vi "TELEOP BUTTONS.vi"(10 "Joystick values":T1(array[cluster])) -> ()   [LabVIEW 2020]
uses:
  <vilib>/Rock Robotics/Network Tables/NT Read Boolean.vi
  <vilib>/Rock Robotics/Network Tables/NT Write Boolean.vi
  <vilib>/Rock Robotics/Network Tables/NT Read Number.vi
  <vilib>/Rock Robotics/Network Tables/NT Read Numeric Array.vi
  <vilib>/Rock Robotics/Network Tables/NT Write Number.vi
panel:
  in  "INTAKE ARM DOWN":cluster{"Joystick":u16, "BUTTON":i32}={"Joystick"=2, "BUTTON"=9} {"Joystick" items=["RIGHT TANK (default)", "LEFT ARM", "RIGHT ARM", "LEFT TANK DRIVE"]}
  in  "FIRE CARGO":cluster{"Joystick":u16, "BUTTON":i32} {"Joystick" items=["RIGHT TANK (default)", "LEFT ARM", "RIGHT ARM", "LEFT TANK DRIVE"]}
  in  "SHOOTER SPEEDS":u16(ring) items=["HI", "LO", "PUKE"]
  in  "SHOOTER off":cluster{"Joystick":u16, "BUTTON":i32}={"Joystick"=2, "BUTTON"=11} {"Joystick" items=["RIGHT TANK (default)", "LEFT ARM", "RIGHT ARM", "LEFT TANK DRIVE"]}
  in  "SHOOTER puke":cluster{"Joystick":u16, "BUTTON":i32}={"Joystick"=2, "BUTTON"=10} {"Joystick" items=["RIGHT TANK (default)", "LEFT ARM", "RIGHT ARM", "LEFT TANK DRIVE"]}
  in  "CLIMBER TURBO":cluster{"Joystick":u16, "BUTTON":i32}={"Joystick"=2, "BUTTON"=9} {"Joystick" items=["RIGHT TANK (default)", "LEFT ARM", "RIGHT ARM", "LEFT TANK DRIVE"]}
  in  "SHOOTER LO":cluster{"Joystick":u16, "BUTTON":i32}={"Joystick"=2, "BUTTON"=8} {"Joystick" items=["RIGHT TANK (default)", "LEFT ARM", "RIGHT ARM", "LEFT TANK DRIVE"]}
  in  "SHOOTER HI":cluster{"Joystick":u16, "BUTTON":i32}={"Joystick"=2, "BUTTON"=7} {"Joystick" items=["RIGHT TANK (default)", "LEFT ARM", "RIGHT ARM", "LEFT TANK DRIVE"]}
  in  "TOGGLE PAWL LOCKS":cluster{"Joystick":u16, "BUTTON":i32}={"Joystick"=2, "BUTTON"=6} {"Joystick" items=["RIGHT TANK (default)", "LEFT ARM", "RIGHT ARM", "LEFT TANK DRIVE"]}
  in  "MACRO LOW BAR CLIMB":cluster{"Joystick":u16, "BUTTON":i32}={"Joystick"=1, "BUTTON"=11} {"Joystick" items=["RIGHT TANK (default)", "LEFT ARM", "RIGHT ARM", "LEFT TANK DRIVE"]}
  in  "INTAKE rollers toggle ON/OFF":cluster{"Joystick":u16, "BUTTON":i32}={"Joystick"=1, "BUTTON"=10} {"Joystick" items=["RIGHT TANK (default)", "LEFT ARM", "RIGHT ARM", "LEFT TANK DRIVE"]}
  in  "INTAKE raise/lower":cluster{"Joystick":u16, "BUTTON":i32}={"Joystick"=1, "BUTTON"=9} {"Joystick" items=["RIGHT TANK (default)", "LEFT ARM", "RIGHT ARM", "LEFT TANK DRIVE"]}
  in  "MACRO overide":cluster{"Joystick":u16, "BUTTON":i32}={"Joystick"=1, "BUTTON"=6} {"Joystick" items=["RIGHT TANK (default)", "LEFT ARM", "RIGHT ARM", "LEFT TANK DRIVE"]}
  in  "MACRO step forward":cluster{"Joystick":u16, "BUTTON":i32}={"Joystick"=1, "BUTTON"=7} {"Joystick" items=["RIGHT TANK (default)", "LEFT ARM", "RIGHT ARM", "LEFT TANK DRIVE"]}
  in  "MACRO step back":cluster{"Joystick":u16, "BUTTON":i32}={"Joystick"=1, "BUTTON"=8} {"Joystick" items=["RIGHT TANK (default)", "LEFT ARM", "RIGHT ARM", "LEFT TANK DRIVE"]}
  in  "AXIS VALUES in":u16(ring) items=["X axis", "Y axis", "Z axis"]
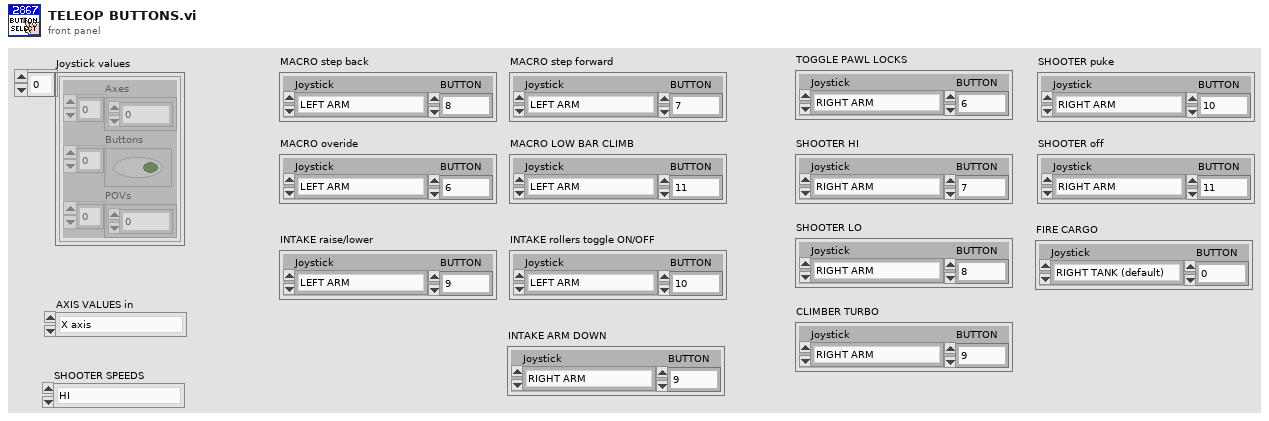
[diagram p1: front panel]
types:
  T1 = cluster{"Axes":dbl[], "Buttons":bool[], "POVs":i16[]}[]
  T2 = cluster{"SHOOTER HI":cluster{"Joystick":u16, "BUTTON":i32}, "SHOOTER puke":cluster{"Joystick":u16, "BUTTON":i32}, "CLIMBER TURBO":cluster{"Joystick":u16, "BUTTON":i32}, "MACRO overide":cluster{"Joystick":u16, "BUTTON":i32}, "TOGGLE PAWL LOCKS":cluster{"Joystick":u16, "BUTTON":i32}, "SHOOTER LO":cluster{"Joystick":u16, "BUTTON":i32}, "MACRO LOW BAR CLIMB":cluster{"Joystick":u16, "BUTTON":i32}, "MACRO step forward":cluster{"Joystick":u16, "BUTTON":i32}, "INTAKE rollers toggle ON/OFF":cluster{"Joystick":u16, "BUTTON":i32}, "MACRO step back":cluster{"Joystick":u16, "BUTTON":i32}, "INTAKE raise/lower":cluster{"Joystick":u16, "BUTTON":i32}, "SHOOTER off":cluster{"Joystick":u16, "BUTTON":i32}, "FIRE CARGO":cluster{"Joystick":u16, "BUTTON":i32}, "INTAKE ARM DOWN":cluster{"Joystick":u16, "BUTTON":i32}}
  T3 = cluster{"Axes":dbl[], "Buttons":bool[], "POVs":i16[]}
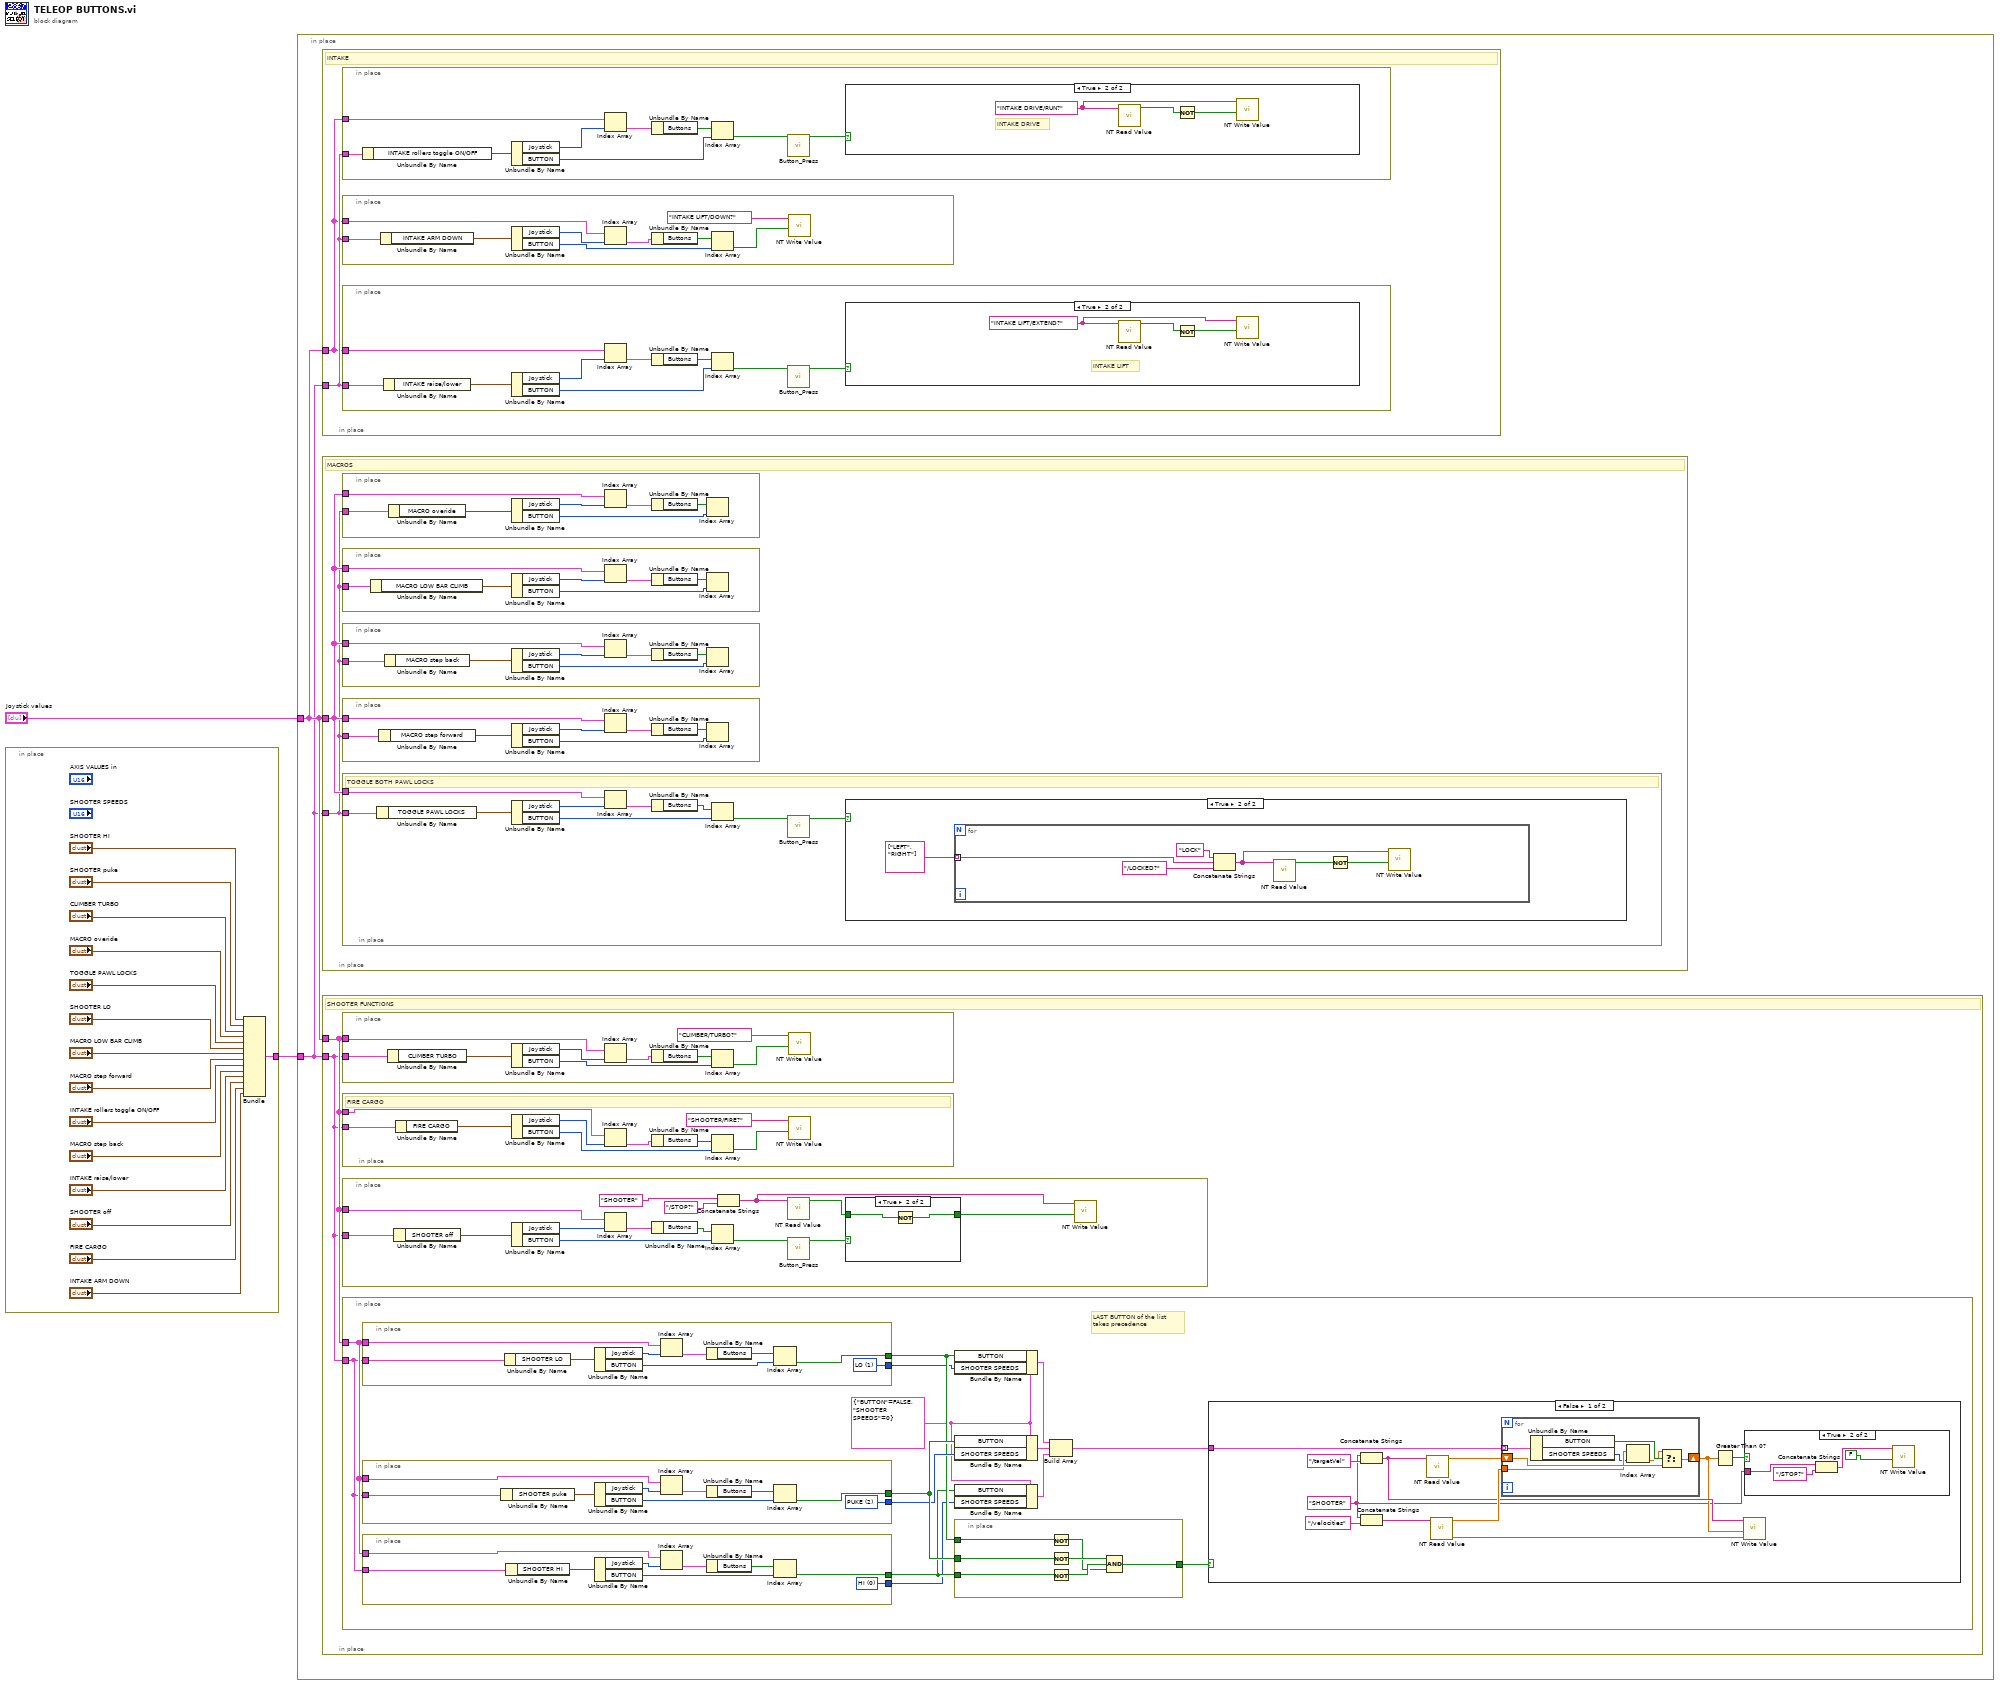
[diagram p0: block diagram]
diagram:
  n1 = in-place {
    in-place-border: [w6] -> w1
    n2 = Bundle("SHOOTER HI"="SHOOTER HI", "SHOOTER puke"="SHOOTER puke", "CLIMBER TURBO"="CLIMBER TURBO", "MACRO overide"="MACRO overide", "TOGGLE PAWL LOCKS"="TOGGLE PAWL LOCKS", "SHOOTER LO"="SHOOTER LO", "MACRO LOW BAR CLIMB"="MACRO LOW BAR CLIMB", "MACRO step forward"="MACRO step forward", "INTAKE rollers toggle ON/OFF"="INTAKE rollers toggle ON/OFF", "MACRO step back"="MACRO step back", "INTAKE raise/lower"="INTAKE raise/lower", "SHOOTER off"="SHOOTER off", "FIRE CARGO"="FIRE CARGO", "INTAKE ARM DOWN"="INTAKE ARM DOWN") -> (w6:T2)  [unwired: 1 in]
  }
  n3 = in-place {
    in-place-border: "Joystick values" -> [w19]
    in-place-border: w1 -> [w18]
    n4 = in-place {
      in-place-border: w19 -> [w173]
      in-place-border: w18 -> [w174]
      # "INTAKE"
      n5 = in-place {
        in-place-border: w173 -> [w192]
        in-place-border: w174 -> [w189]
        n6 = Unbundle By Name(w189) -> ("INTAKE rollers toggle ON/OFF"=w188:cluster{"Joystick":u16, "BUTTON":i32})
        n7 = Unbundle By Name(w188) -> ("Joystick"=w187:u16, "BUTTON"=w186:i32)
        n8 = Index Array(array=w192, index=w187) -> (element=w191:T3)
        n9 = Unbundle By Name(w191) -> ("Buttons"=w190:bool[])
        n10 = Index Array(array=w190, index=w186) -> (element=w184:bool)
        n11 = call "Button_Press.vi"("Button In"=w184) -> ("Button Pressed?"=w185:bool)  [unwired: 10 in]
        n12 = case shown="True" w185 {
          frame False {
          }
          frame True {
            w193 = "INTAKE DRIVE/RUN?" ("Name")
            # "INTAKE DRIVE"
            n13 = call-poly <vilib>:"NT Read Value.vi"("Name"=w193) -> ("Boolean"=w195:bool)  [unwired: 9 in, 1 out]
            n14 = Not(x=w195) -> (.not. x?=w194:bool)
            n15 = call-poly <vilib>:"NT Write Value.vi"("Boolean"=w194, "Name"=w193) -> ()  [unwired: 9 in, 1 out]
          }
        }
      }
      n16 = in-place {
        in-place-border: w173 -> [w183]
        in-place-border: w174 -> [w180]
        n17 = Unbundle By Name(w180) -> ("INTAKE ARM DOWN"=w179:cluster{"Joystick":u16, "BUTTON":i32})
        n18 = Unbundle By Name(w179) -> ("Joystick"=w178:u16, "BUTTON"=w177:i32)
        n19 = Index Array(array=w183, index=w178) -> (element=w182:T3)
        n20 = Unbundle By Name(w182) -> ("Buttons"=w181:bool[])
        n21 = Index Array(array=w181, index=w177) -> (element=w175:bool)
        n22 = call-poly <vilib>:"NT Write Value.vi"("Boolean"=w175, "Name"="INTAKE LIFT/DOWN?") -> ()  [unwired: 9 in, 1 out]
      }
      n23 = in-place {
        in-place-border: w173 -> [w204]
        in-place-border: w174 -> [w201]
        n24 = Unbundle By Name(w201) -> ("INTAKE raise/lower"=w200:cluster{"Joystick":u16, "BUTTON":i32})
        n25 = Unbundle By Name(w200) -> ("Joystick"=w199:u16, "BUTTON"=w198:i32)
        n26 = Index Array(array=w204, index=w199) -> (element=w203:T3)
        n27 = Unbundle By Name(w203) -> ("Buttons"=w202:bool[])
        n28 = Index Array(array=w202, index=w198) -> (element=w197:bool)
        n29 = call "Button_Press.vi"("Button In"=w197) -> ("Button Pressed?"=w196:bool)  [unwired: 10 in]
        n30 = case shown="True" w196 {
          frame False {
          }
          frame True {
            w205 = "INTAKE LIFT/EXTEND?" ("Name")
            # "INTAKE LIFT"
            n31 = call-poly <vilib>:"NT Read Value.vi"("Name"=w205) -> ("Boolean"=w207:bool)  [unwired: 9 in, 1 out]
            n32 = Not(x=w207) -> (.not. x?=w206:bool)
            n33 = call-poly <vilib>:"NT Write Value.vi"("Boolean"=w206, "Name"=w205) -> ()  [unwired: 9 in, 1 out]
          }
        }
      }
    }
    n34 = in-place {
      in-place-border: w19 -> [w128]
      in-place-border: w18 -> [w127]
      # "MACROS"
      n35 = in-place {
        in-place-border: w128 -> [w165]
        in-place-border: w127 -> [w162]
        n36 = Unbundle By Name(w162) -> ("MACRO overide"=w161:cluster{"Joystick":u16, "BUTTON":i32})
        n37 = Unbundle By Name(w161) -> ("Joystick"=w160:u16, "BUTTON"=w159:i32)
        n38 = Index Array(array=w165, index=w160) -> (element=w164:T3)
        n39 = Unbundle By Name(w164) -> ("Buttons"=w163:bool[])
        n40 = Index Array(array=w163, index=w159) -> ()  [unwired: 1 out]
      }
      n41 = in-place {
        in-place-border: w128 -> [w172]
        in-place-border: w127 -> [w169]
        n42 = Unbundle By Name(w169) -> ("MACRO LOW BAR CLIMB"=w168:cluster{"Joystick":u16, "BUTTON":i32})
        n43 = Unbundle By Name(w168) -> ("Joystick"=w167:u16, "BUTTON"=w166:i32)
        n44 = Index Array(array=w172, index=w167) -> (element=w171:T3)
        n45 = Unbundle By Name(w171) -> ("Buttons"=w170:bool[])
        n46 = Index Array(array=w170, index=w166) -> ()  [unwired: 1 out]
      }
      n47 = in-place {
        in-place-border: w128 -> [w158]
        in-place-border: w127 -> [w155]
        n48 = Unbundle By Name(w155) -> ("MACRO step back"=w154:cluster{"Joystick":u16, "BUTTON":i32})
        n49 = Unbundle By Name(w154) -> ("Joystick"=w153:u16, "BUTTON"=w152:i32)
        n50 = Index Array(array=w158, index=w153) -> (element=w157:T3)
        n51 = Unbundle By Name(w157) -> ("Buttons"=w156:bool[])
        n52 = Index Array(array=w156, index=w152) -> ()  [unwired: 1 out]
      }
      n53 = in-place {
        in-place-border: w128 -> [w151]
        in-place-border: w127 -> [w148]
        n54 = Unbundle By Name(w148) -> ("MACRO step forward"=w147:cluster{"Joystick":u16, "BUTTON":i32})
        n55 = Unbundle By Name(w147) -> ("Joystick"=w146:u16, "BUTTON"=w145:i32)
        n56 = Index Array(array=w151, index=w146) -> (element=w150:T3)
        n57 = Unbundle By Name(w150) -> ("Buttons"=w149:bool[])
        n58 = Index Array(array=w149, index=w145) -> ()  [unwired: 1 out]
      }
      n59 = in-place {
        in-place-border: w128 -> [w137]
        in-place-border: w127 -> [w134]
        # "TOGGLE BOTH PAWL LOCKS"
        n60 = Unbundle By Name(w134) -> ("TOGGLE PAWL LOCKS"=w133:cluster{"Joystick":u16, "BUTTON":i32})
        n61 = Unbundle By Name(w133) -> ("Joystick"=w132:u16, "BUTTON"=w131:i32)
        n62 = Index Array(array=w137, index=w132) -> (element=w136:T3)
        n63 = Unbundle By Name(w136) -> ("Buttons"=w135:bool[])
        n64 = Index Array(array=w135, index=w131) -> (element=w129:bool)
        n65 = call "Button_Press.vi"("Button In"=w129) -> ("Button Pressed?"=w130:bool)  [unwired: 10 in]
        n66 = case shown="True" w130 {
          frame False {
          }
          frame True {
            n67 = for {
              tunnel: string[] ["LEFT", "RIGHT"] -> [w139] mode=indexing
              n68 = Concatenate Strings("LOCK" ("string"), w139, "/LOCKED?" ("Name")) -> (w141:string)
              n69 = call-poly <vilib>:"NT Read Value.vi"("Name"=w141) -> ("Boolean"=w144:bool)  [unwired: 9 in, 1 out]
              n70 = Not(x=w144) -> (.not. x?=w143:bool)
              n71 = call-poly <vilib>:"NT Write Value.vi"("Boolean"=w143, "Name"=w141) -> ()  [unwired: 9 in, 1 out]
            }
          }
        }
      }
    }
    n72 = in-place {
      in-place-border: w19 -> [w21]
      in-place-border: w18 -> [w20]
      # "SHOOTER FUNCTIONS"
      n73 = in-place {
        in-place-border: w21 -> [w100]
        in-place-border: w20 -> [w97]
        n74 = Unbundle By Name(w97) -> ("CLIMBER TURBO"=w96:cluster{"Joystick":u16, "BUTTON":i32})
        n75 = Unbundle By Name(w96) -> ("Joystick"=w95:u16, "BUTTON"=w94:i32)
        n76 = Index Array(array=w100, index=w95) -> (element=w99:T3)
        n77 = Unbundle By Name(w99) -> ("Buttons"=w98:bool[])
        n78 = Index Array(array=w98, index=w94) -> (element=w93:bool)
        n79 = call-poly <vilib>:"NT Write Value.vi"("Boolean"=w93, "Name"="CLIMBER/TURBO?") -> ()  [unwired: 9 in, 1 out]
      }
      n80 = in-place {
        in-place-border: w21 -> [w102]
        in-place-border: w20 -> [w103]
        # "FIRE CARGO"
        n81 = Unbundle By Name(w103) -> ("FIRE CARGO"=w107:cluster{"Joystick":u16, "BUTTON":i32})
        n82 = Unbundle By Name(w107) -> ("Joystick"=w106:u16, "BUTTON"=w105:i32)
        n83 = Index Array(array=w102, index=w106) -> (element=w109:T3)
        n84 = Unbundle By Name(w109) -> ("Buttons"=w108:bool[])
        n85 = Index Array(array=w108, index=w105) -> (element=w101:bool)
        n86 = call-poly <vilib>:"NT Write Value.vi"("Boolean"=w101, "Name"="SHOOTER/FIRE?") -> ()  [unwired: 9 in, 1 out]
      }
      n87 = in-place {
        in-place-border: w21 -> [w123]
        in-place-border: w20 -> [w120]
        n88 = Unbundle By Name(w120) -> ("SHOOTER off"=w119:cluster{"Joystick":u16, "BUTTON":i32})
        n89 = Unbundle By Name(w119) -> ("Joystick"=w118:u16, "BUTTON"=w117:i32)
        n90 = Index Array(array=w123, index=w118) -> (element=w122:T3)
        n91 = Unbundle By Name(w122) -> ("Buttons"=w121:bool[])
        n92 = Index Array(array=w121, index=w117) -> (element=w114:bool)
        n93 = Concatenate Strings("SHOOTER", "/STOP?" ("string")) -> (w113:string)
        n94 = call-poly <vilib>:"NT Read Value.vi"("Name"=w113) -> ("Boolean"=w112:bool)  [unwired: 9 in, 1 out]
        n95 = call "Button_Press.vi"("Button In"=w114) -> ("Button Pressed?"=w110:bool)  [unwired: 10 in]
        n96 = case shown="True" w110 {
          tunnel: w112 -> [w124 w126]
          tunnel: [w124 w125] -> w111
          frame False {
          }
          frame True {
            n97 = Not(x=w126) -> (.not. x?=w125:bool)
          }
        }
        n98 = call-poly <vilib>:"NT Write Value.vi"("Boolean"=w111, "Name"=w113) -> ()  [unwired: 9 in, 1 out]
      }
      n99 = in-place {
        in-place-border: w21 -> [w35]
        in-place-border: w20 -> [w34]
        w28 = cluster{"BUTTON":bool, "SHOOTER SPEEDS":u16} {"BUTTON"=FALSE, "SHOOTER SPEEDS"=0}
        # "LAST BUTTON of the list\ntakes precedence"
        n100 = in-place {
          in-place-border: w35 -> [w91]
          in-place-border: w34 -> [w88]
          in-place-border: [w84] -> w29
          in-place-border: [w83] -> w30
          w84 = u16 1 items=["HI", "LO", "PUKE"] ("SHOOTER SPEEDS")
          n101 = Unbundle By Name(w88) -> ("SHOOTER LO"=w87:cluster{"Joystick":u16, "BUTTON":i32})
          n102 = Unbundle By Name(w87) -> ("Joystick"=w86:u16, "BUTTON"=w85:i32)
          n103 = Index Array(array=w91, index=w86) -> (element=w90:T3)
          n104 = Unbundle By Name(w90) -> ("Buttons"=w89:bool[])
          n105 = Index Array(array=w89, index=w85) -> (element=w83:bool)
        }
        n106 = in-place {
          in-place-border: w35 -> [w82]
          in-place-border: w34 -> [w79]
          in-place-border: [w75] -> w32
          in-place-border: [w74] -> w31
          w74 = u16 2 items=["HI", "LO", "PUKE"] ("SHOOTER SPEEDS")
          n107 = Unbundle By Name(w79) -> ("SHOOTER puke"=w78:cluster{"Joystick":u16, "BUTTON":i32})
          n108 = Unbundle By Name(w78) -> ("Joystick"=w77:u16, "BUTTON"=w76:i32)
          n109 = Index Array(array=w82, index=w77) -> (element=w81:T3)
          n110 = Unbundle By Name(w81) -> ("Buttons"=w80:bool[])
          n111 = Index Array(array=w80, index=w76) -> (element=w75:bool)
        }
        n112 = in-place {
          in-place-border: w35 -> [w73]
          in-place-border: w34 -> [w70]
          in-place-border: [w66] -> w27
          in-place-border: [w65] -> w26
          w65 = u16 0 items=["HI", "LO", "PUKE"] ("SHOOTER SPEEDS")
          n113 = Unbundle By Name(w70) -> ("SHOOTER HI"=w69:cluster{"Joystick":u16, "BUTTON":i32})
          n114 = Unbundle By Name(w69) -> ("Joystick"=w68:u16, "BUTTON"=w67:i32)
          n115 = Index Array(array=w73, index=w68) -> (element=w72:T3)
          n116 = Unbundle By Name(w72) -> ("Buttons"=w71:bool[])
          n117 = Index Array(array=w71, index=w67) -> (element=w66:bool)
        }
        n118 = Bundle By Name(cluster=w28, "BUTTON"=w30, "SHOOTER SPEEDS"=w29) -> (w25:cluster{"BUTTON":bool, "SHOOTER SPEEDS":u16})
        n119 = Bundle By Name(cluster=w28, "BUTTON"=w32, "SHOOTER SPEEDS"=w31) -> (w24:cluster{"BUTTON":bool, "SHOOTER SPEEDS":u16})
        n120 = Bundle By Name(cluster=w28, "BUTTON"=w27, "SHOOTER SPEEDS"=w26) -> (w23:cluster{"BUTTON":bool, "SHOOTER SPEEDS":u16})
        n121 = in-place {
          in-place-border: w32 -> [w42]
          in-place-border: w27 -> [w41]
          in-place-border: w30 -> [w40]
          in-place-border: [w36] -> w33
          n122 = Not(x=w40) -> (.not. x?=w37:bool)
          n123 = Not(x=w42) -> (.not. x?=w39:bool)
          n124 = Not(x=w41) -> (.not. x?=w38:bool)
          n125 = Compound Arithmetic op=AND(w39, w38, w37) -> (w36:bool)
        }
        n126 = Build Array(w25, w24, w23) -> (w22:cluster{"BUTTON":bool, "SHOOTER SPEEDS":u16}[])
        n127 = case shown="False" w33 {
          tunnel: w22 -> [w53 _]
          frame False {
            w43 = "SHOOTER"
            n128 = Concatenate Strings(w43, "/targetVel" ("string")) -> (w47:string)
            n129 = Concatenate Strings(w43, "/velocities" ("Name")) -> (w50:string)
            n130 = call-poly <vilib>:"NT Read Value.vi"("Name"=w47) -> ("Numeric"=w46:dbl)  [unwired: 9 in, 1 out]
            n131 = call-poly <vilib>:"NT Read Value.vi"("Name"=w50) -> ("error out"=w49:errorcluster, "Numeric Array"=w48:dbl[])  [unwired: 9 in]
            n132 = for {
              tunnel: w53 -> [w63] mode=indexing
              tunnel: w48 -> [w60]
              shift-right: [w62] -> w45
              shift-left: w46 -> [w64]
              n133 = Unbundle By Name(w63) -> ("BUTTON"=w61:bool, "SHOOTER SPEEDS"=w59:u16)
              n134 = Index Array(array=w60, index=w59) -> (element=w58:dbl)
              n135 = Select(t=w58, s=w61, f=w64) -> (s? t:f=w62:dbl)
            }
            n136 = Greater Than 0?(x=w45) -> (x > 0?=w44:bool)
            n137 = call-poly <vilib>:"NT Write Value.vi"("error in"=w49, "Numeric"=w45, "Name"=w47) -> ()  [unwired: 8 in, 1 out]
            n138 = case shown="True" w44 {
              tunnel: w43 -> [_ w56]
              frame False {
              }
              frame True {
                n139 = Concatenate Strings(w56, "/STOP?" ("string")) -> (w55:string)
                n140 = call-poly <vilib>:"NT Write Value.vi"("Boolean"=FALSE, "Name"=w55) -> ()  [unwired: 9 in, 1 out]
              }
            }
          }
          frame True {
          }
        }
      }
    }
  }
